vi "Send_message_from_UI_to_ConrtolLoop.vi"(5 "data DVR in":refnum<data-value>, 11 "error in (no error)":errorcluster, 12 "timeout in ms (10)":i32=45000) -> (15 "error out":errorcluster)   [LabVIEW 2019, in "Service.lvlib"]
uses:
  Service.lvlib
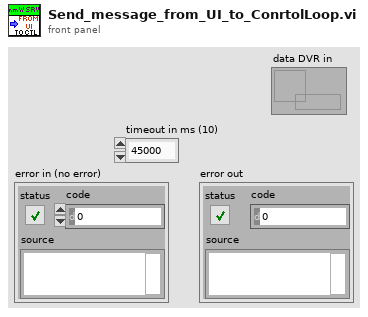
[diagram p1: front panel]
types:
  T1 = typedef "Service.lvlib/AppData.ctl" = cluster{"MsgQ":refnum<queue>, "Stop?":bool, "zmq sessions":cluster{"Control_endpoint":string, "Instr_endpoint":string}, "control-loop":cluster{"fromUI-Q":refnum<queue>, "toUI":refnum<user-event>, "Control_endpoint":string}, "UI-loop":cluster{"evnt_ref":refnum<event-registration>}, "logging":cluster{"level":dbl, "verbosity":dbl, "path":string, "Listener_ID":string}, "general_settings":cluster{"mmW_instr_ini_path":string, "mmW_instr_pid_path":string}}
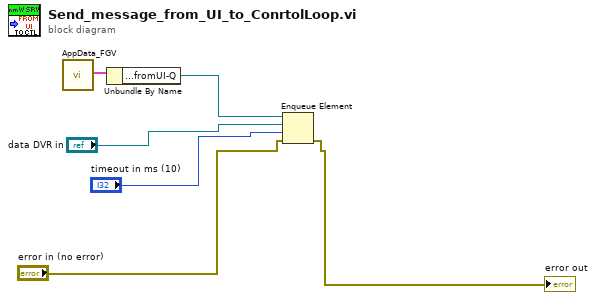
[diagram p0: block diagram]
diagram:
  n1 = call "AppData_FGV.vi"() -> ("AppData out"=w6:T1)  [unwired: 18 in, 1 out]
  n2 = Unbundle By Name(w6) -> ("control-loop.fromUI-Q"=w5:refnum<queue>)
  n3 = Enqueue Element(queue=w5, element="data DVR in", timeout in ms (-1)="timeout in ms (10)", error in (no error)="error in (no error)") -> (error out=→"error out":errorcluster)  [unwired: 2 out]
